vi "通用New.vi"(8 "error in (no error)":errorcluster caption="错误输入（无错误）", 10 "通用配置":T1={"ModBusRTU反馈"=enum."无反馈", "侦听周期"=0, "跳转反馈"=FALSE, "报文记录数量"=0, "客服端新增模式"=enum."单端模式"}, 11 "MainPage 输入":refnum<class "MainPage.lvclass">) -> (0 "error out":errorcluster caption="错误输出", 3 "MainPage 输出":refnum<class "MainPage.lvclass">)   [LabVIEW 2019, in "MainPage.lvlib" / "MainPage.lvclass"]
uses:
  MainPage.lvclass
  MainPage.lvclass/MainPage.ctl
panel:
  out "通用引用":refnum<data-value>
  # "实际+10ms间隔时间"
  # "达到上限会顶替旧记录"
  # "实际+10ms间隔时间"
  # "达到上限会顶替旧记录"
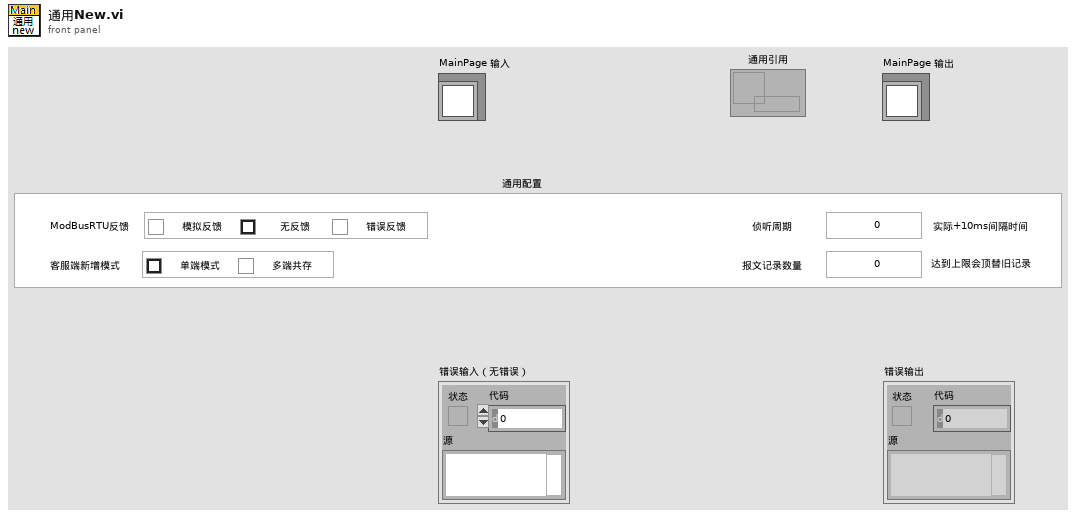
[diagram p1: front panel]
types:
  T1 = typedef "MainPage.lvlib/MainPage.lvclass/通用配置选项.ctl" = cluster{"ModBusRTU反馈":enum32{"模拟反馈", "无反馈", "错误反馈"}, "侦听周期":u32, "跳转反馈":bool, "报文记录数量":u16, "客服端新增模式":enum32{"单端模式", "多端共存"}}
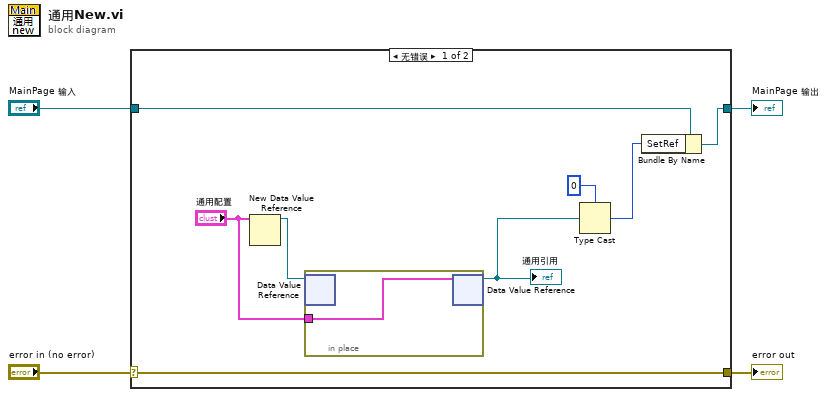
[diagram p0: block diagram]
diagram:
  n1 = case shown="无错误" "error in (no error)" {
    selector: "error in (no error)" -> [w12 w15]
    tunnel: [w12 w15] -> w3
    tunnel: [w8 w14] -> w1
    tunnel: "MainPage 输入" -> [w10 w14]
    frame No Error {
      n2 = New Data Value Reference(data value="通用配置") -> (data value reference=w6:refnum<data-value>)  [unwired: 1 in, 1 out]
      n3 = in-place {
        in-place-border: "通用配置" -> [w13]
        n4 = in-place-dvr #1(w6) -> ()  [unwired: 2 out]
        n5 = in-place-dvr #1(w13) -> (w5:refnum<data-value>)  [unwired: 1 out]
      }
      "通用引用" <- w5
      n6 = Type Cast(type=u32 0 ("DataRef"), x=w5) -> (*(type *) &x=w9:u32)
      n7 = Bundle By Name(cluster=w10, "SetRef"=w9) -> (w8:refnum<class "MainPage.lvclass">)
    }
    frame Error {
    }
  }
  "error out" <- w3
  "MainPage 输出" <- w1
